vi "FTW-ERR-Clear.vi"(1 "error to snuff":errorcluster) -> (0 "no error":errorcluster)   [LabVIEW 2013, in "XML.lvlib"]
uses:
  XML.lvlib
panel:
  # "Inputs"
  # "Outputs"
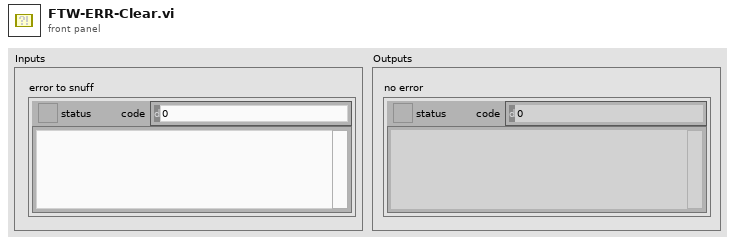
[diagram p1: front panel]
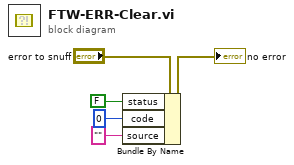
[diagram p0: block diagram]
diagram:
  n1 = Bundle By Name(cluster="error to snuff", "status"=FALSE, "code"=0, "source"="") -> (→"no error":errorcluster)
